vi "StepRun.vi"(5 "EndTime":timestamp, 7 "StartTime":timestamp, 8 "error in":errorcluster, 11 "StepRun":refnum<class "StepRun.lvclass">) -> (0 "error out":errorcluster, 3 "Passed":bool)   [LabVIEW 2020]
uses:
  <vilib>/Averna/ProligentResultProcessor/ProligentResultProcessor.lvlibp/StepRun/StepRun/StepRun.lvclass
  <vilib>/Averna/ProligentResultProcessor/ProligentResultProcessor.lvlibp/StepRun/StepRun/SetStepName.vi
  <vilib>/Averna/ProligentResultProcessor/ProligentResultProcessor.lvlibp/StepRun/StepRun/SetStepExecutionStatus.vi
  <vilib>/Averna/ProligentResultProcessor/ProligentResultProcessor.lvlibp/StepRun/StepRun/SetStartDate.vi
  <vilib>/Averna/ProligentResultProcessor/ProligentResultProcessor.lvlibp/StepRun/StepRun/SetEndDate.vi
  <vilib>/Averna/ProligentResultProcessor/ProligentResultProcessor.lvlibp/StepRun/StepRun/SetStepRunId.vi
  <vilib>/Averna/ProligentResultProcessor/ProligentResultProcessor.lvlibp/StepRun/StepRun/GetStepName.vi
  <vilib>/Averna/ProligentResultProcessor/ProligentResultProcessor.lvlibp/StepRun/StepRun/GetStepExecutionStatus.vi
  <vilib>/Averna/ProligentResultProcessor/ProligentResultProcessor.lvlibp/StepRun/StepRun/GetStartDate.vi
  <vilib>/Averna/ProligentResultProcessor/ProligentResultProcessor.lvlibp/StepRun/StepRun/GetEndDate.vi
  <vilib>/Averna/ProligentResultProcessor/ProligentResultProcessor.lvlibp/StepRun/StepRun/GetStepRunId.vi
  <vilib>/Averna/ProligentResultProcessor/ProligentResultProcessor.lvlibp/StepRun/StepRun/GetMeasures.vi
  <vilib>/Averna/ProligentResultProcessor/ProligentResultProcessor.lvlibp/StepRun/StepRun/GetCharacteristics.vi
  <vilib>/Averna/ProligentResultProcessor/ProligentResultProcessor.lvlibp/StepRun/StepRun/GetDocuments.vi
  <vilib>/Averna/ProligentResultProcessor/ProligentResultProcessor.lvlibp/StepRun/StepRun/GetFailureReferences.vi
  <vilib>/Averna/ProligentResultProcessor/ProligentResultProcessor.lvlibp/StepRun/StepRun/GetCustomData.vi
  <vilib>/Averna/ProligentResultProcessor/ProligentResultProcessor.lvlibp/Measure/Measure/Measure.lvclass
  <vilib>/Averna/ProligentResultProcessor/ProligentResultProcessor.lvlibp/Model/Characteristic/Characteristic.lvclass
  <vilib>/Averna/ProligentResultProcessor/ProligentResultProcessor.lvlibp/Model/Document/Document.lvclass
  <vilib>/Averna/ProligentResultProcessor/ProligentResultProcessor.lvlibp/Failure/FailureReference/FailureReference.lvclass
  <vilib>/Averna/ProligentResultProcessor/ProligentResultProcessor.lvlibp/Model/CustomData/CustomData.lvclass
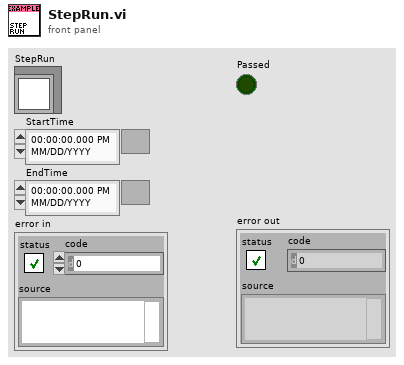
[diagram p1: front panel]
types:
  T1 = enum16{"PASS", "FAIL", "NOT_COMPLETED", "ABORTED"}
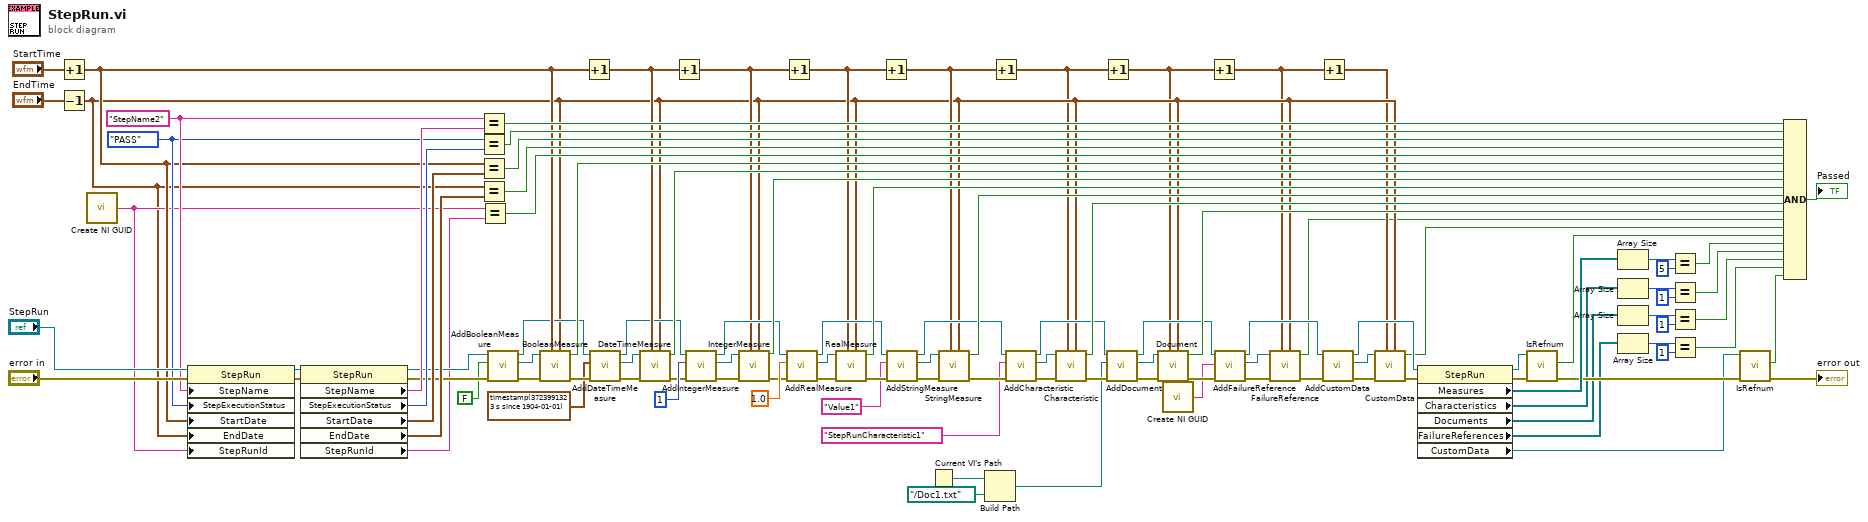
[diagram p0: block diagram]
diagram:
  w78 = T1."PASS" ("ProcessRunStatus")
  w89 = "StepName2"
  n1 = Increment(x="StartTime") -> (x+1=w56:timestamp)
  n2 = Decrement(x="EndTime") -> (x-1=w11:timestamp)
  n3 = call <vilib>:"Create NI GUID.vi"() -> ("NI GUID"=w29:string)
  n4 = property class="StepRun"(reference="StepRun", error in="error in", "StepName"=w89, "StepExecutionStatus"=w78, "StartDate"=w56, "EndDate"=w11, "StepRunId"=w29) -> (reference out=w95:refnum<class "StepRun.lvclass">, error out=w94:errorcluster)
  n5 = property class="StepRun"(reference=w95, error in=w94) -> (reference out=w88:refnum<class "StepRun.lvclass">, error out=w87:errorcluster, "StepName"=w93:string, "StepExecutionStatus"=w92:T1, "StartDate"=w91:timestamp, "EndDate"=w90:timestamp, "StepRunId"=w30:string)
  n6 = Equal?(x=w89, y=w93) -> (x = y?=w108:bool)
  n7 = Equal?(x=w78, y=w92) -> (x = y?=w107:bool)
  n8 = Equal?(x=w56, y=w91) -> (x = y?=w106:bool)
  n9 = Equal?(x=w11, y=w90) -> (x = y?=w110:bool)
  n10 = Equal?(x=w29, y=w30) -> (x = y?=w109:bool)
  n11 = call <vilib>:"AddBooleanMeasure.vi"("error in"=w87, "Value"=FALSE, "StepRun in"=w88) -> ("error out"=w75:errorcluster, "BooleanMeasure"=w76:refnum<class "BooleanMeasure.lvclass">, "StepRun out"=w53:refnum<class "StepRun.lvclass">)  [unwired: 6 in]
  n12 = call "BooleanMeasure.vi"("EndTime"=w11, "StartTime"=w56, "error in"=w75, "BooleanMeasure"=w76) -> ("error out"=w63:errorcluster, "Passed"=w104:bool)  [unwired: 6 in]
  n13 = Increment(x=w56) -> (x+1=w55:timestamp)
  n14 = call <vilib>:"AddDateTimeMeasure.vi"("error in"=w63, "Value"=timestamp(3723991323.456 s since 1904-01-01), "StepRun in"=w53) -> ("error out"=w58:errorcluster, "RealMeasure"=w54:refnum<class "DateTimeMeasure.lvclass">, "StepRun out"=w52:refnum<class "StepRun.lvclass">)  [unwired: 6 in]
  n15 = call "DateTimeMeasure.vi"("EndTime"=w11, "StartTime"=w55, "error in"=w58, "DateTimeMeasure"=w54) -> ("error out"=w57:errorcluster, "Passed"=w100:bool)  [unwired: 6 in]
  n16 = Increment(x=w55) -> (x+1=w64:timestamp)
  n17 = call <vilib>:"AddIntegerMeasure.vi"("error in"=w57, "Value"=i64 1, "StepRun in"=w52) -> ("error out"=w68:errorcluster, "RealMeasure"=w67:refnum<class "IntegerMeasure.lvclass">, "StepRun out"=w66:refnum<class "StepRun.lvclass">)  [unwired: 6 in]
  n18 = call "IntegerMeasure.vi"("EndTime"=w11, "StartTime"=w64, "error in"=w68, "IntegerlMeasure"=w67) -> ("error out"=w65:errorcluster, "Passed"=w102:bool)  [unwired: 6 in]
  n19 = Increment(x=w64) -> (x+1=w49:timestamp)
  n20 = call <vilib>:"AddRealMeasure.vi"("error in"=w65, "Value"=1.0, "StepRun in"=w66) -> ("error out"=w72:errorcluster, "RealMeasure"=w71:refnum<class "RealMeasure.lvclass">, "StepRun out"=w59:refnum<class "StepRun.lvclass">)  [unwired: 6 in]
  n21 = call "RealMeasure.vi"("EndTime"=w11, "StartTime"=w49, "error in"=w72, "RealMeasure"=w71) -> ("error out"=w62:errorcluster, "Passed"=w103:bool)  [unwired: 6 in]
  n22 = Increment(x=w49) -> (x+1=w12:timestamp)
  n23 = call <vilib>:"AddStringMeasure.vi"("error in"=w62, "Value"="Value1", "StepRun in"=w59) -> ("error out"=w50:errorcluster, "StringMeasure"=w51:refnum<class "StringMeasure.lvclass">, "StepRun out"=w35:refnum<class "StepRun.lvclass">)  [unwired: 6 in]
  n24 = Current VI's Path() -> (path=w3:path)
  n25 = call "StringMeasure.vi"("EndTime"=w11, "StartTime"=w12, "error in"=w50, "StringMeasure"=w51) -> ("error out"=w39:errorcluster, "Passed"=w101:bool)  [unwired: 6 in]
  n26 = Build Path(base path=w3, name or relative path=path "../Doc1.txt") -> (appended path=w2:path)
  n27 = Increment(x=w12) -> (x+1=w9:timestamp)
  n28 = call <vilib>:"AddCharacteristic.vi"("error in"=w39, "FullName"="StepRunCharacteristic1", "StepRun in"=w35) -> ("error out"=w38:errorcluster, "Characteristic"=w36:refnum<class "Characteristic.lvclass">, "StepRun out"=w32:refnum<class "StepRun.lvclass">)  [unwired: 6 in]
  n29 = call "Characteristic.vi"("EndTime"=w11, "StartTime"=w9, "error in (no error)"=w38, "Characteristic in"=w36) -> ("error out"=w37:errorcluster, "Passed"=w99:bool)  [unwired: 6 in]
  n30 = Increment(x=w9) -> (x+1=w8:timestamp)
  n31 = call <vilib>:"AddDocument.vi"("error in"=w37, "FilePath"=w2, "StepRun in"=w32) -> ("error out"=w33:errorcluster, "Document"=w31:refnum<class "Document.lvclass">, "StepRun out"=w26:refnum<class "StepRun.lvclass">)  [unwired: 6 in]
  n32 = call "Document.vi"("EndTime"=w11, "StartTime"=w8, "error in (no error)"=w33, "Document in"=w31) -> ("error out"=w28:errorcluster, "Passed"=w98:bool)  [unwired: 6 in]
  n33 = call <vilib>:"Create NI GUID.vi"() -> ("NI GUID"=w10:string)
  n34 = Increment(x=w8) -> (x+1=w7:timestamp)
  n35 = call <vilib>:"AddFailureReference.vi"("error in"=w28, "Id"=w10, "StepRun in"=w26) -> ("error out"=w27:errorcluster, "FailureReference"=w24:refnum<class "FailureReference.lvclass">, "StepRun out"=w16:refnum<class "StepRun.lvclass">)  [unwired: 6 in]
  n36 = call "FailureReference.vi"("EndTime"=w11, "StartTime"=w7, "error in"=w27, "FailureReference"=w24) -> ("error out"=w25:errorcluster, "Passed"=w5:bool)  [unwired: 6 in]
  n37 = Increment(x=w7) -> (x+1=w6:timestamp)
  n38 = call <vilib>:"AddCustomData.vi"("error in (no error)"=w25, "StepRun in"=w16) -> ("error out"=w17:errorcluster, "CustomData"=w13:refnum<class "CustomData.lvclass">, "StepRun out"=w15:refnum<class "StepRun.lvclass">)  [unwired: 7 in]
  n39 = call "CustomData.vi"("EndTime"=w11, "StartTime"=w6, "error in"=w17, "CustomData"=w13) -> ("error out"=w14:errorcluster, "Passed"=w4:bool)  [unwired: 6 in]
  n40 = property class="StepRun"(reference=w15, error in=w14) -> (reference out=w73:refnum<class "StepRun.lvclass">, error out=w83:errorcluster, "Measures"=w84:refnum<class "Measure.lvclass">[], "Characteristics"=w23:refnum<class "Characteristic.lvclass">[], "Documents"=w22:refnum<class "Document.lvclass">[], "FailureReferences"=w21:refnum<class "FailureReference.lvclass">[], "CustomData"=w19:refnum<class "CustomData.lvclass">)
  n41 = call <vilib>:"IsRefnum.vi"("error in"=w83, "StepRun in"=w73) -> ("error out"=w74:errorcluster, "IsRefnum"=w105:bool)  [unwired: 7 in, 1 out]
  n42 = Array Size(array=w84) -> (size(s)=w86:i32)
  n43 = Array Size(array=w23) -> (size(s)=w47:i32)
  n44 = Array Size(array=w22) -> (size(s)=w46:i32)
  n45 = Array Size(array=w21) -> (size(s)=w43:i32)
  n46 = Equal?(x=w86, y=5) -> (x = y?=w82:bool)
  n47 = Equal?(x=w47, y=1) -> (x = y?=w42:bool)
  n48 = Equal?(x=w46, y=1) -> (x = y?=w41:bool)
  n49 = Equal?(x=w43, y=1) -> (x = y?=w40:bool)
  n50 = call <vilib>:"IsRefnum.vi"("error in"=w74, "CustomDataType in"=w19) -> ("error out"=→"error out":errorcluster, "IsRefnum"=w18:bool)  [unwired: 7 in, 1 out]
  n51 = Compound Arithmetic op=AND(w108, w107, w106, w110, w109, w104, w100, w102, w103, w101, w99, w98, w5, w4, w105, w82, w42, w41, w40, w18) -> (→"Passed":bool)
